vi "GUI.vi"() -> ()   [LabVIEW 2020]
uses:
  <vilib>/DAQmx/write.llb/DAQmx Write (Analog 1D DBL NChan 1Samp).vi
  <vilib>/DAQmx/create/channels.llb/DAQmx Create Channel (AO-Voltage-Basic).vi
  <vilib>/DAQmx/miscellaneous.llb/DAQmx Fill In Error Info.vi
panel:
  in  "Shutter":bool
  in  "Power (%)":dbl(slide)=100.0 scale=0.0..100.0
  out "Emitting:":bool=TRUE
  in  "stop":bool
  # "Analog control AOMs Salix"
  # "515 nm"
  # "561 nm"
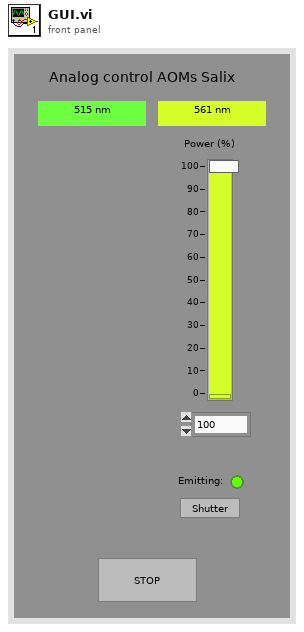
[diagram p1: front panel]
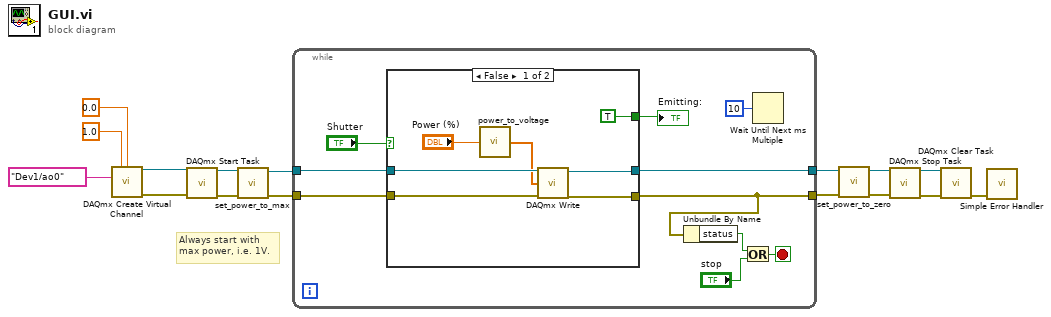
[diagram p0: block diagram]
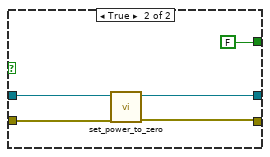
[diagram p2: hidden frame]
diagram:
  # "Always start with\nmax power, i.e. 1V."
  n1 = call-poly <vilib>:"DAQmx Create Virtual Channel.vi"("maximum value"=1.0, "minimum value"=0.0, "physical channels"=tag "Dev1/ao0") -> ("task out"=w13:refnum<k21>, "error out"=w12:errorcluster)  [unwired: 11 in]
  n2 = call <vilib>:"DAQmx Start Task.vi"("task/channels in"=w13, "error in"=w12) -> ("task out"=w4:refnum<k21>, "error out"=w3:errorcluster)  [unwired: 12 in]
  n3 = call "set_power_to_max.vi"("error in"=w3, "task/channels in"=w4) -> ("error out"=w1:errorcluster, "task out"=w2:refnum<k21>)  [unwired: 8 in]
  n4 = while {
    tunnel: w2 -> [w25]
    tunnel: w1 -> [w24]
    tunnel: [w22] -> w6
    tunnel: [w21] -> w7
    stop <- w26 stop-if-true
    n5 = case shown="False" "Shutter" {
      tunnel: w25 -> [w33 w37]
      tunnel: w24 -> [w32 w35]
      tunnel: [w31 w34] -> w22
      tunnel: [w30 w36] -> w21
      tunnel: [TRUE ("Boolean") FALSE ("Boolean")] -> w18
      frame False {
        n6 = call "power_to_voltage.vi"("Power (%)"="Power (%)") -> ("Voltage"=w29:dbl[])
        n7 = call-poly <vilib>:"DAQmx Write.vi"("task/channels in"=w33, "data"=w29, "error in"=w32) -> ("task out"=w30:refnum<k21>, "error out"=w31:errorcluster)  [unwired: 10 in, 1 out]
      }
      frame True {
        n8 = call "set_power_to_zero.vi"("error in"=w35, "task/channels in"=w37) -> ("error out"=w34:errorcluster, "task out"=w36:refnum<k21>)  [unwired: 8 in]
      }
    }
    "Emitting:" <- w18
    n9 = Unbundle By Name(w22) -> ("status"=w23:bool)
    n10 = Or(x=w23, y="stop") -> (x .or. y?=w26:bool)
    n11 = Wait Until Next ms Multiple(millisecond multiple=u32 10) -> ()  [unwired: 1 out]
  }
  n12 = call "set_power_to_zero.vi"("error in"=w6, "task/channels in"=w7) -> ("error out"=w8:errorcluster, "task out"=w9:refnum<k21>)  [unwired: 8 in]
  n13 = call <vilib>:"DAQmx Stop Task.vi"("task/channels in"=w9, "error in"=w8) -> ("task out"=w16:refnum<k21>, "error out"=w15:errorcluster)  [unwired: 12 in]
  n14 = call <vilib>:"DAQmx Clear Task.vi"("task in"=w16, "error in"=w15) -> ("error out"=w14:errorcluster)  [unwired: 13 in]
  n15 = call <vilib>:"Simple Error Handler.vi"("error in (no error)"=w14) -> ()  [unwired: 4 in, 5 out]
